vi "Read Transactions.vi"(8 "error in (no error)":errorcluster, 11 "Simulated User Console Actor in":refnum<class "Simulated User Console Actor.lvclass">) -> (0 "error out":errorcluster, 2 "Transactions":refnum<vi>, 3 "Simulated User Console Actor out":refnum<class "Simulated User Console Actor.lvclass">)   [LabVIEW 2019, in "Simulated User Console Actor.lvlib" / "Simulated User Console Actor.lvclass"]
uses:
  Simulated User Console Actor.lvclass
  Transactions -Cluster.ctl
  Simulated User Console Actor.lvclass/Simulated User Console Actor.ctl
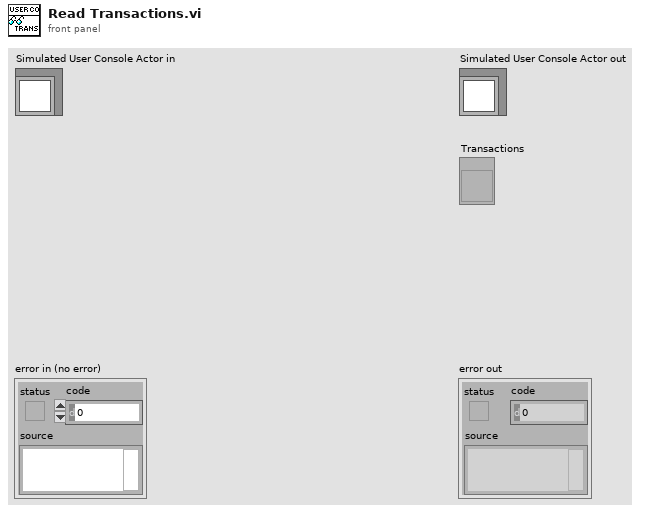
[diagram p1: front panel]
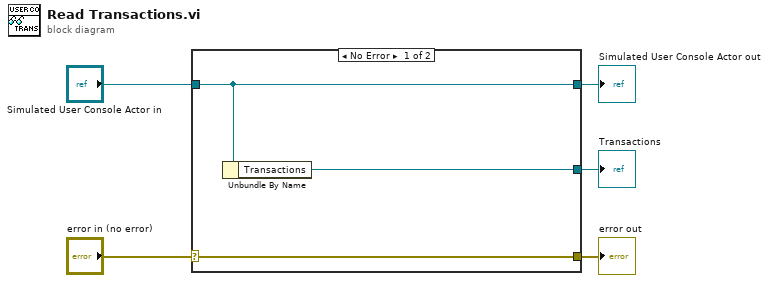
[diagram p0: block diagram]
diagram:
  n1 = case shown="No Error" "error in (no error)" {
    selector: "error in (no error)" -> [w8 w9]
    tunnel: [w8 w9] -> w4
    tunnel: [w7 w10] -> w2
    tunnel: "Simulated User Console Actor in" -> [w7 w10]
    tunnel: [w6 _] -> w1
    frame No Error {
      n2 = Unbundle By Name(w7) -> ("Transactions"=w6:refnum<vi>)
    }
    frame Error {
    }
  }
  "error out" <- w4
  "Simulated User Console Actor out" <- w2
  "Transactions" <- w1
